vi "Client_Side.vi"() -> ()   [LabVIEW 2021]
panel:
  in  "Panel Control":T1(tab)
  in  "Enter":bool
  out "Please Enter your Pincode to login?":string
  in  "clear":bool
  in  "cancel":bool
  in  "7":bool
  in  "8":bool
  in  "9":bool
  in  "1":bool
  in  "2":bool
  in  "3":bool
  in  "4":bool
  in  "5":bool
  in  "6":bool
  in  "0":bool
  in  "Bedroom-1 Door":dbl(slide) scale=0.0..2.0
  in  "Bedroom-1 Light":bool
  in  "Bedroom-1 Curtains":dbl(knob) scale=0.0..9.0
  in  "Bedroom-2 Door":dbl(slide) scale=0.0..2.0
  in  "Bedroom-2 Light":bool
  in  "Bedroom-2 Curtains":dbl(knob) scale=0.0..9.0
  in  "Master Light":bool
  in  "Master Curtains":dbl(knob) scale=0.0..9.0
  in  "Master Door":dbl(slide) scale=0.0..2.0
  in  "Volume":dbl(slide) scale=0.0..9.0
  in  "Turn TV On/Off":bool
  in  "Channel":u32 min=1 max=5
  in  "Living Room Curtains":dbl(knob) scale=0.0..9.0
  in  "Living Room Light":bool
  in  "Living Room Door":dbl(slide) scale=0.0..2.0
  in  "Balcony Light - 2":bool
  in  "Balcony Light - 1":bool
  in  "Balcony Light - 3":bool
  in  "Kitchen Curtains":dbl(knob) scale=0.0..9.0
  in  "Kitchen Light":bool
  in  "Kitchen Door":dbl(slide) scale=0.0..2.0
  # "Bedroom - 1"
  # "Bedroom - 2"
  # "Master Bedroom"
  # "Living Room"
  # "Balcony"
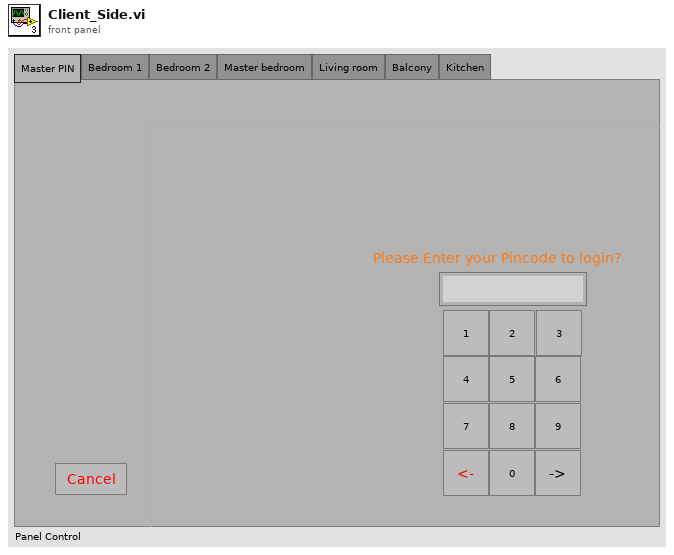
[diagram p1: front panel]
types:
  T1 = enum32{"Master PIN", "Bedroom 1", "Bedroom 2", "Master bedroom", "Living room", "Balcony", "Kitchen"}
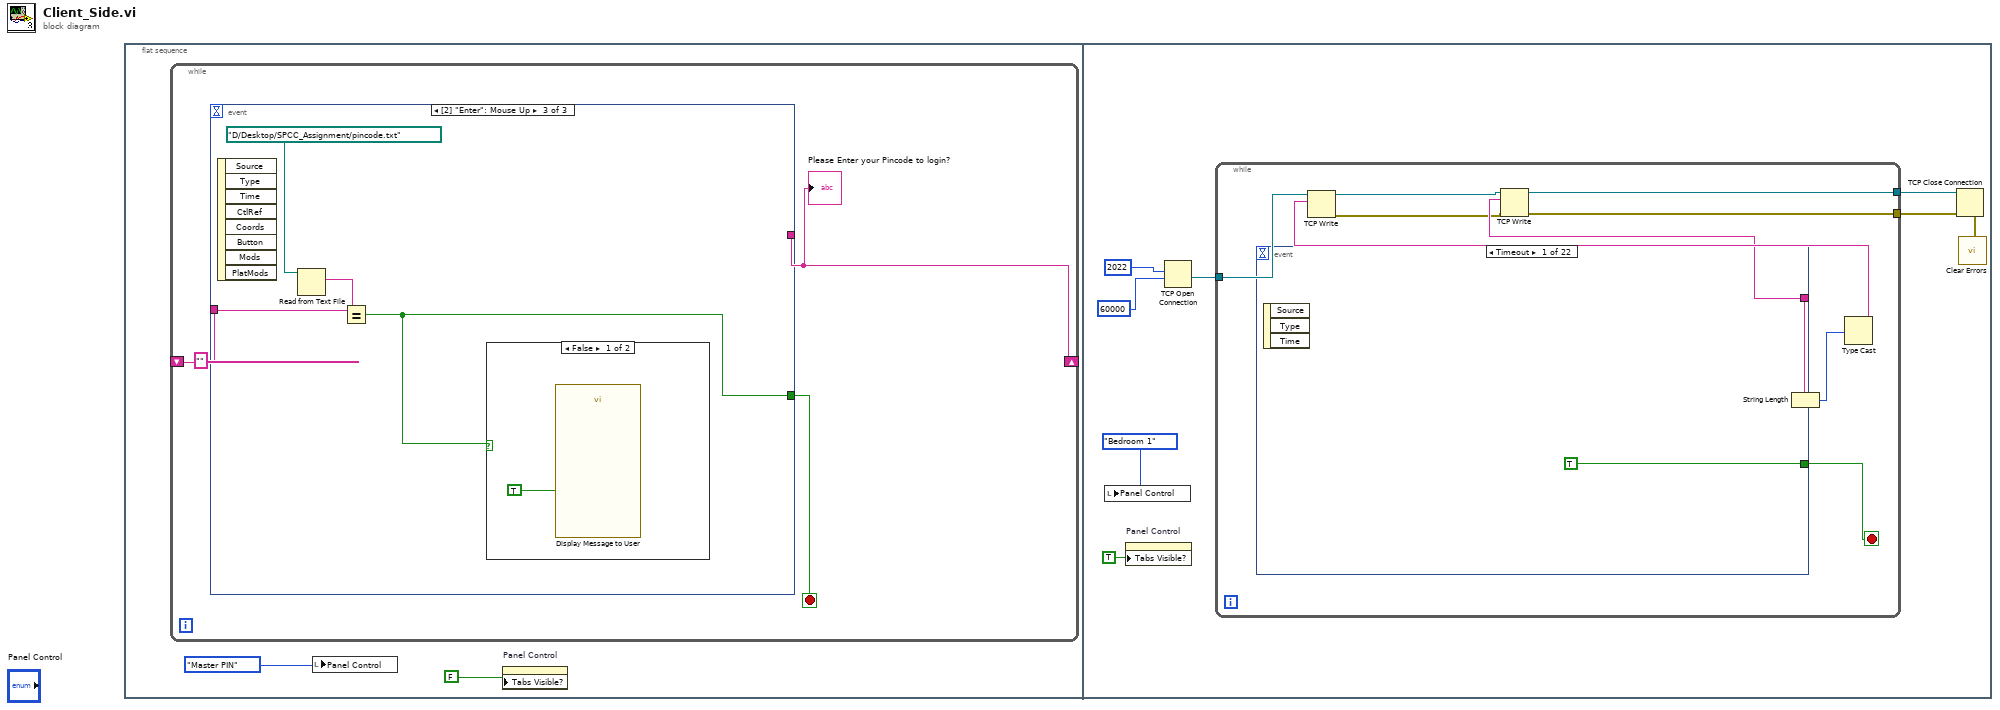
[diagram p0: block diagram]
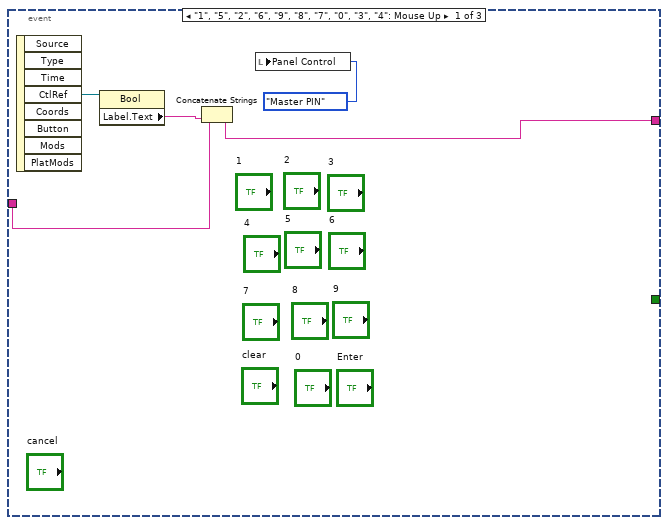
[diagram p2: hidden frame]
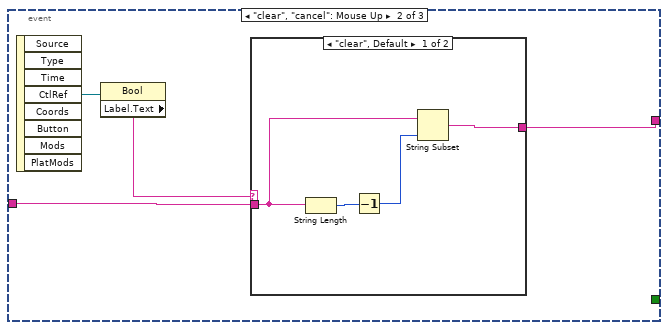
[diagram p3: hidden frame]
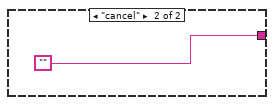
[diagram p4: hidden frame]
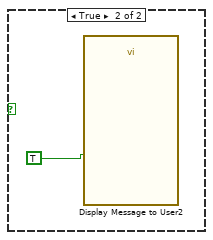
[diagram p5: hidden frame]
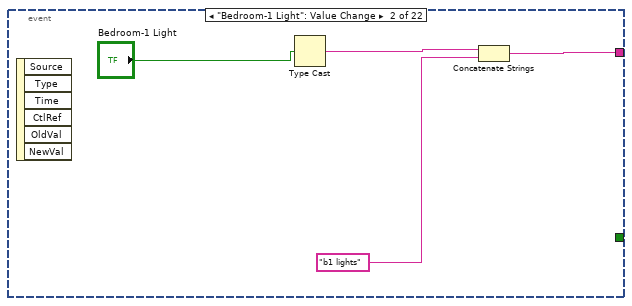
[diagram p6: hidden frame]
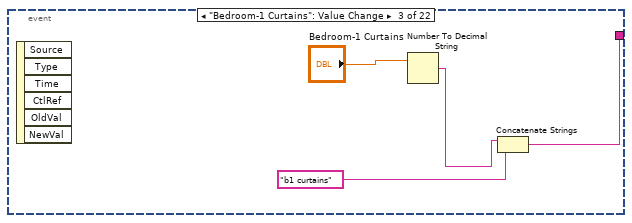
[diagram p7: hidden frame]
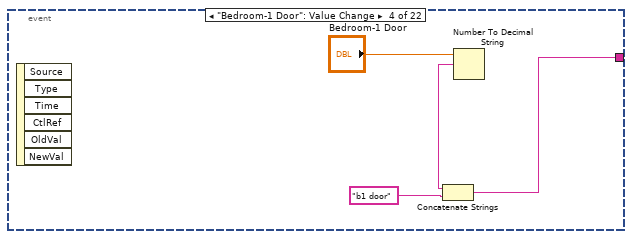
[diagram p8: hidden frame]
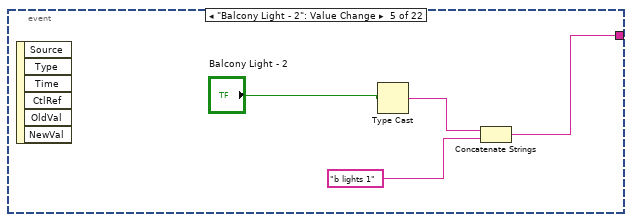
[diagram p9: hidden frame]
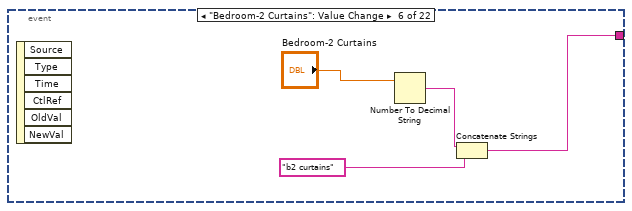
[diagram p10: hidden frame]
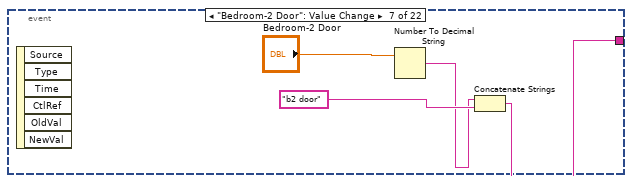
[diagram p11: hidden frame]
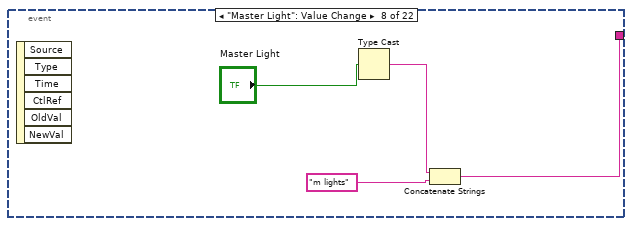
[diagram p12: hidden frame]
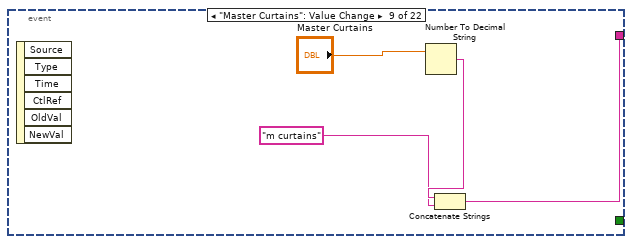
[diagram p13: hidden frame]
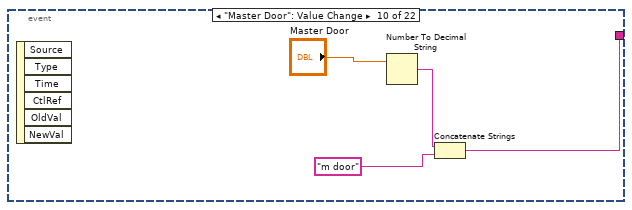
[diagram p14: hidden frame]
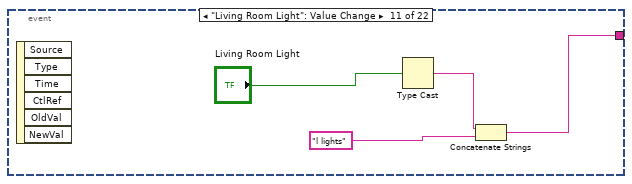
[diagram p15: hidden frame]
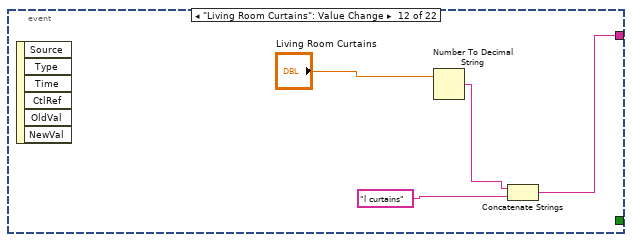
[diagram p16: hidden frame]
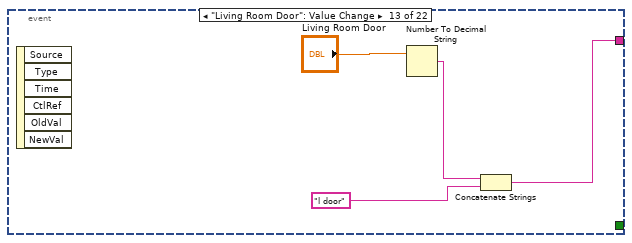
[diagram p17: hidden frame]
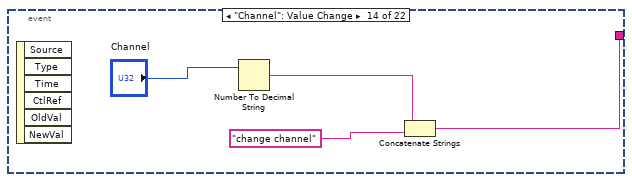
[diagram p18: hidden frame]
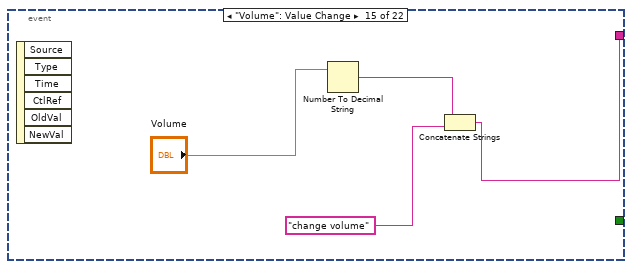
[diagram p19: hidden frame]
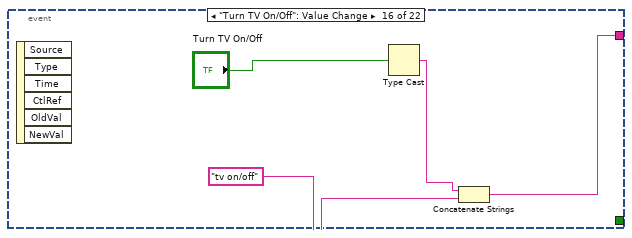
[diagram p20: hidden frame]
diagram:
  n1 = flat-sequence {
    frame #0 {
      n2 = while {
        shift-right: [w5] -> _
        shift-left: "" -> [w6]
        stop <- w4 stop-if-true
        n3 = event shown="[2] \"Enter\": Mouse Up" {
          selector: _ -> [_ _ _]
          dyn-events: _ -> [_ _ _]
          timeout: _ -> [_ _ _]
          tunnel: w6 -> [w9 w13 w23]
          tunnel: [w8 w12 _] -> w5
          tunnel: [_ _ w21] -> w4
          event "1", "5", "2", "6", "9", "8", "7", "0", "3", "4": Mouse Up {
            n4 = event-data() -> ("CtlRef"=w11:refnum<vi>)  [unwired: 1 in, 7 out]
            n5 = property class="Bool"(reference=w11) -> ("Label.Text"=w10:string)  [unwired: 1 in, 2 out]
            n6 = Concatenate Strings(w9, w10) -> (w8:string)
            n7 = local write "Panel Control"(T1."Master PIN" ("Tab Control")) -> ()
          }
          event "clear", "cancel": Mouse Up {
            n8 = event-data() -> ("CtlRef"=w15:refnum<vi>)  [unwired: 1 in, 7 out]
            n9 = property class="Bool"(reference=w15) -> ("Label.Text"=w14:string)  [unwired: 1 in, 2 out]
            n10 = case shown="\"clear\", Default" w14 {
              tunnel: w13 -> [w17 _]
              tunnel: [w16 ""] -> w12
              frame "clear", Default {
                n11 = String Length(string=w17) -> (length=w18:i32)
                n12 = Decrement(x=w18) -> (x-1=w19:i32)
                n13 = String Subset(string=w17, length (rest)=w19) -> (substring=w16:string)  [unwired: 1 in]
              }
              frame "cancel" {
              }
            }
          }
          event "Enter": Mouse Up {
            n14 = event-data() -> ()  [unwired: 1 in, 8 out]
            n15 = Read from Text File(file (use dialog)=path "D:/Desktop/SPCC_Assignment/pincode.txt") -> (text=w22:string)  [unwired: 3 in, 3 out]
            n16 = Equal?(x=w23, y=w22) -> (x = y?=w21:bool)
            n17 = case shown="False" w21 {
              frame False {
                n18 = call "Display Message to User"("Enable"=TRUE) -> ()  [unwired: 9 in, 2 out]
              }
              frame True {
                n19 = call "Display Message to User2"("Enable"=TRUE) -> ()  [unwired: 9 in, 2 out]
              }
            }
          }
        }
        "Please Enter your Pincode to login?" <- w5
      }
      n20 = local write "Panel Control"(T1."Master PIN" ("Tab Control")) -> ()
      n21 = property on="Panel Control" class="TabCtl (strict)"("Tabs Visible?"=FALSE) -> ()  [unwired: 2 in, 2 out]
    }
    frame #1 {
      n22 = local write "Panel Control"(T1."Bedroom 1" ("Tab Control")) -> ()
      n23 = property on="Panel Control" class="TabCtl (strict)"("Tabs Visible?"=TRUE) -> ()  [unwired: 2 in, 2 out]
      n24 = TCP Open Connection(remote port or service name=2022, timeout ms (60000)=60000) -> (connection ID=w32:refnum<k5>)  [unwired: 3 in, 1 out]
      n25 = while {
        tunnel: w32 -> [w43]
        tunnel: [w38] -> w31
        tunnel: [w36] -> w30
        stop <- w37 stop-if-true
        n26 = event shown="[0] Timeout" {
          selector: _ -> [_ _ _ _ _ _ _ _ _ _ _ _ _ _ _ _ _ _ _ _ _ _]
          dyn-events: _ -> [_ _ _ _ _ _ _ _ _ _ _ _ _ _ _ _ _ _ _ _ _ _]
          timeout: _ -> [_ _ _ _ _ _ _ _ _ _ _ _ _ _ _ _ _ _ _ _ _ _]
          tunnel: [_ w48 w51 w56 w57 w62 w67 w69 w73 w79 w81 w85 w89 w93 w98 w101 w105 w111 w113 w117 w121 w126] -> w39
          tunnel: [TRUE _ _ _ _ _ _ _ _ _ _ _ _ _ _ _ _ _ _ _ _ _] -> w37
          event Timeout {
            n27 = event-data() -> ()  [unwired: 1 in, 3 out]
          }
          event "Bedroom-1 Light": Value Change {
            n28 = event-data() -> ()  [unwired: 1 in, 6 out]
            n29 = Type Cast(x="Bedroom-1 Light") -> (*(type *) &x=w46:string)  [unwired: 1 in]
            n30 = Concatenate Strings "Concatenate Strings"(w46, "b1 lights") -> (w48:string)
          }
          event "Bedroom-1 Curtains": Value Change {
            n31 = event-data() -> ()  [unwired: 1 in, 6 out]
            n32 = Number To Decimal String(number="Bedroom-1 Curtains") -> (decimal integer string=w50:string)  [unwired: 1 in]
            n33 = Concatenate Strings "Concatenate Strings"(w50, "b1 curtains") -> (w51:string)
          }
          event "Bedroom-1 Door": Value Change {
            n34 = event-data() -> ()  [unwired: 1 in, 6 out]
            n35 = Number To Decimal String(number="Bedroom-1 Door") -> (decimal integer string=w53:string)  [unwired: 1 in]
            n36 = Concatenate Strings "Concatenate Strings"(w53, "b1 door") -> (w56:string)
          }
          event "Balcony Light - 2": Value Change {
            n37 = event-data() -> ()  [unwired: 1 in, 6 out]
            n38 = Type Cast(x="Balcony Light - 2") -> (*(type *) &x=w59:string)  [unwired: 1 in]
            n39 = Concatenate Strings "Concatenate Strings"(w59, "b lights 1") -> (w57:string)
          }
          event "Bedroom-2 Curtains": Value Change {
            n40 = event-data() -> ()  [unwired: 1 in, 6 out]
            n41 = Number To Decimal String(number="Bedroom-2 Curtains") -> (decimal integer string=w64:string)  [unwired: 1 in]
            n42 = Concatenate Strings "Concatenate Strings"(w64, "b2 curtains") -> (w62:string)
          }
          event "Bedroom-2 Door": Value Change {
            n43 = event-data() -> ()  [unwired: 1 in, 6 out]
            n44 = Number To Decimal String(number="Bedroom-2 Door") -> (decimal integer string=w66:string)  [unwired: 1 in]
            n45 = Concatenate Strings "Concatenate Strings"(w66, "b2 door") -> (w67:string)
          }
          event "Master Light": Value Change {
            n46 = event-data() -> ()  [unwired: 1 in, 6 out]
            n47 = Type Cast(x="Master Light") -> (*(type *) &x=w72:string)  [unwired: 1 in]
            n48 = Concatenate Strings "Concatenate Strings"(w72, "m lights") -> (w69:string)
          }
          event "Master Curtains": Value Change {
            n49 = event-data() -> ()  [unwired: 1 in, 6 out]
            n50 = Number To Decimal String(number="Master Curtains") -> (decimal integer string=w76:string)  [unwired: 1 in]
            n51 = Concatenate Strings "Concatenate Strings"(w76, "m curtains") -> (w73:string)
          }
          event "Master Door": Value Change {
            n52 = event-data() -> ()  [unwired: 1 in, 6 out]
            n53 = Number To Decimal String(number="Master Door") -> (decimal integer string=w78:string)  [unwired: 1 in]
            n54 = Concatenate Strings "Concatenate Strings"(w78, "m door") -> (w79:string)
          }
          event "Living Room Light": Value Change {
            n55 = event-data() -> ()  [unwired: 1 in, 6 out]
            n56 = Type Cast(x="Living Room Light") -> (*(type *) &x=w83:string)  [unwired: 1 in]
            n57 = Concatenate Strings "Concatenate Strings"(w83, "l lights") -> (w81:string)
          }
          event "Living Room Curtains": Value Change {
            n58 = event-data() -> ()  [unwired: 1 in, 6 out]
            n59 = Number To Decimal String(number="Living Room Curtains") -> (decimal integer string=w88:string)  [unwired: 1 in]
            n60 = Concatenate Strings "Concatenate Strings"(w88, "l curtains") -> (w85:string)
          }
          event "Living Room Door": Value Change {
            n61 = event-data() -> ()  [unwired: 1 in, 6 out]
            n62 = Number To Decimal String(number="Living Room Door") -> (decimal integer string=w92:string)  [unwired: 1 in]
            n63 = Concatenate Strings "Concatenate Strings"(w92, "l door") -> (w89:string)
          }
          event "Channel": Value Change {
            n64 = event-data() -> ()  [unwired: 1 in, 6 out]
            n65 = Number To Decimal String(number="Channel") -> (decimal integer string=w94:string)  [unwired: 1 in]
            n66 = Concatenate Strings "Concatenate Strings"(w94, "change channel") -> (w93:string)
          }
          event "Volume": Value Change {
            n67 = event-data() -> ()  [unwired: 1 in, 6 out]
            n68 = Number To Decimal String(number="Volume") -> (decimal integer string=w99:string)  [unwired: 1 in]
            n69 = Concatenate Strings "Concatenate Strings"(w99, "change volume") -> (w98:string)
          }
          event "Turn TV On/Off": Value Change {
            n70 = event-data() -> ()  [unwired: 1 in, 6 out]
            n71 = Type Cast(x="Turn TV On/Off") -> (*(type *) &x=w104:string)  [unwired: 1 in]
            n72 = Concatenate Strings "Concatenate Strings"(w104, "tv on/off") -> (w101:string)
          }
          event "Kitchen Light": Value Change {
            n73 = event-data() -> ()  [unwired: 1 in, 6 out]
            n74 = Type Cast(x="Kitchen Light") -> (*(type *) &x=w107:string)  [unwired: 1 in]
            n75 = Concatenate Strings "Concatenate Strings"(w107, "k lights") -> (w105:string)
          }
          event "Kitchen Door": Value Change {
            n76 = event-data() -> ()  [unwired: 1 in, 6 out]
            n77 = Number To Decimal String(number="Kitchen Door") -> (decimal integer string=w109:string)  [unwired: 1 in]
            n78 = Concatenate Strings "Concatenate Strings"(w109, "k door") -> (w111:string)
          }
          event "Kitchen Curtains": Value Change {
            n79 = event-data() -> ()  [unwired: 1 in, 6 out]
            n80 = Number To Decimal String(number="Kitchen Curtains") -> (decimal integer string=w116:string)  [unwired: 1 in]
            n81 = Concatenate Strings "Concatenate Strings"(w116, "k curtains") -> (w113:string)
          }
          event "Balcony Light - 1": Value Change {
            n82 = event-data() -> ()  [unwired: 1 in, 6 out]
            n83 = Type Cast(x="Balcony Light - 1") -> (*(type *) &x=w120:string)  [unwired: 1 in]
            n84 = Concatenate Strings "Concatenate Strings"(w120, "b lights 2") -> (w117:string)
          }
          event "Balcony Light - 3": Value Change {
            n85 = event-data() -> ()  [unwired: 1 in, 6 out]
            n86 = Type Cast(x="Balcony Light - 3") -> (*(type *) &x=w124:string)  [unwired: 1 in]
            n87 = Concatenate Strings "Concatenate Strings"(w124, "b lights 3") -> (w121:string)
          }
          event "Bedroom-2 Light": Value Change {
            n88 = event-data() -> ()  [unwired: 1 in, 6 out]
            n89 = Type Cast(x="Bedroom-2 Light") -> (*(type *) &x=w128:string)  [unwired: 1 in]
            n90 = Concatenate Strings "Concatenate Strings"(w128, "b2 lights") -> (w126:string)
          }
        }
        n91 = String Length(string=w39) -> (length=w42:i32)
        n92 = Type Cast(x=w42) -> (*(type *) &x=w41:string)  [unwired: 1 in]
        n93 = TCP Write(connection ID=w43, data in=w41) -> (connection ID out=w40:refnum<k5>, error out=w35:errorcluster)  [unwired: 2 in, 1 out]
        n94 = TCP Write(connection ID=w40, data in=w39, error in (no error)=w35) -> (connection ID out=w38:refnum<k5>, error out=w36:errorcluster)  [unwired: 1 in, 1 out]
      }
      n95 = TCP Close Connection(connection ID=w31, error in (no error)=w30) -> (error out=w29:errorcluster)  [unwired: 1 in, 1 out]
      n96 = call <vilib>:"Clear Errors.vi"("error in (no error)"=w29) -> ()  [unwired: 5 in, 2 out]
    }
  }
